vi "Modul Reset.vi"(1 "Maximale Beschleunigung":i32=500 min=0 max=2047 step=1, 2 "Mikro-Schrittweite":i32=6 min=0 max=6 step=1, 3 "maximale Positionierungsgeschwindigkeit":i32=115 min=0 max=2047 step=1, 4 "maximaler Strom [mA]":i32=700 min=0 max=1500 step=1, 5 "flow control":u16(ring) items=["None"=0, "XON/XOFF"=1, "RTS/CTS"=2, "DTR/DSR"=4], 6 "VISA resource name":refnum<visa-resource-name>="COM5", 7 "stop bits":u16(ring)=10 items=["1.0"=10, "1.5"=15, "2.0"=20], 8 "parity":u16(ring) items=["None", "Odd", "Even", "Mark", "Space"], 9 "data bits":u16=8 min=5 max=8 step=1, 10 "baud rate":u32=9600) -> (0 "Fehler":bool)   [LabVIEW 2019]
doc: "Die VI \"Modul Reset\" schickt eine Reihe von Befehlen an das Modul TMCM-110 das an eine Serielle Schnittstelle angeschlossen sein muss. Diese setzen und speichern die werte für:\n-maximale Positioniergeschwindigkeit\n-Mikro-Schrittweite\n-maximale Beschleunigung\n-maximaler Strom [mA]\nDie Werte für den Motor sind für die Verwendung mit dem Drehmagnetometer voreingestellt und müssen daher nicht notwendigerweise beschrieben werden.\nEs ist nur darauf zu achten, dass die Adresse der seriellen RS232 Schnittstelle korrekt ist."
uses:
  <vilib>/Instr/_visa.llb/VISA Configure Serial Port (Serial Instr).vi
panel:
  out "Value":string="00"
  out "Motor":string="00"
  out "Instruction":string="1E"
  out "Data to write":string="011E01000020"
  out "Type":string="01"
  # "Durch das Durchführen dieser VI wird die aktuelle Motorposition mit der Nullposition belegt.\nDes weiteren werden die Werte für die Schrittweite und die Positionierungsgeschwindigkeit\nüberschrieben und gespeichert.\nIm Frontpanel müssen nur die Werte für die Serielle Schnittstelle korrekt eingegben werden."
  # "Daten für Schnittstelle"
  # "Daten, die an den Motor geschickt werden (live)"
  # "In den Motor zu schreibende Daten"
  # "Leuchtet diese Lampe auf kann der Motor nicht ausgelesen werden!\nFolgende Ursachen sind möglich:\n-Motor hat keinen Strom\n-Motor ist nicht angeschlossen\n-RS232 Konfigurationen sind falsch"
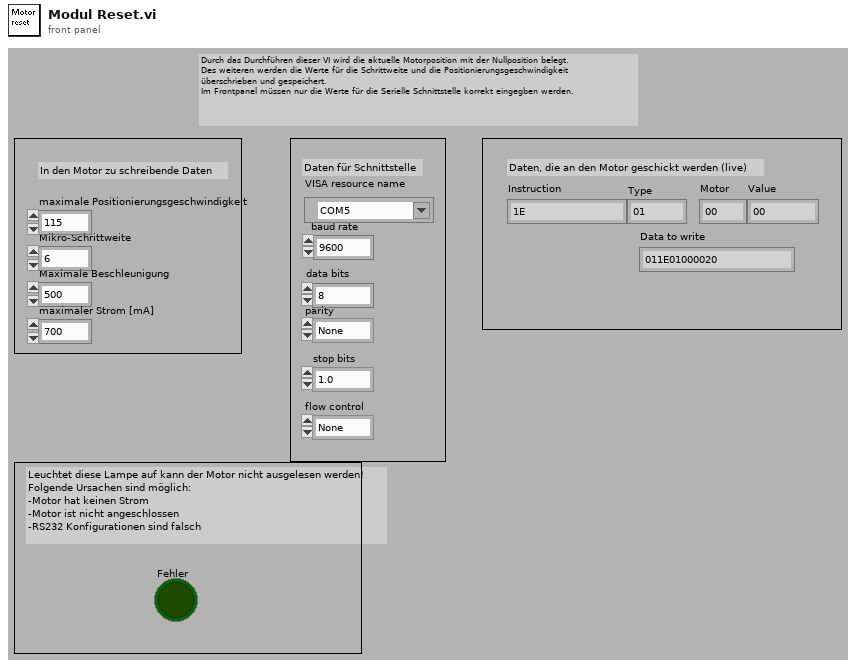
[diagram p1: front panel]
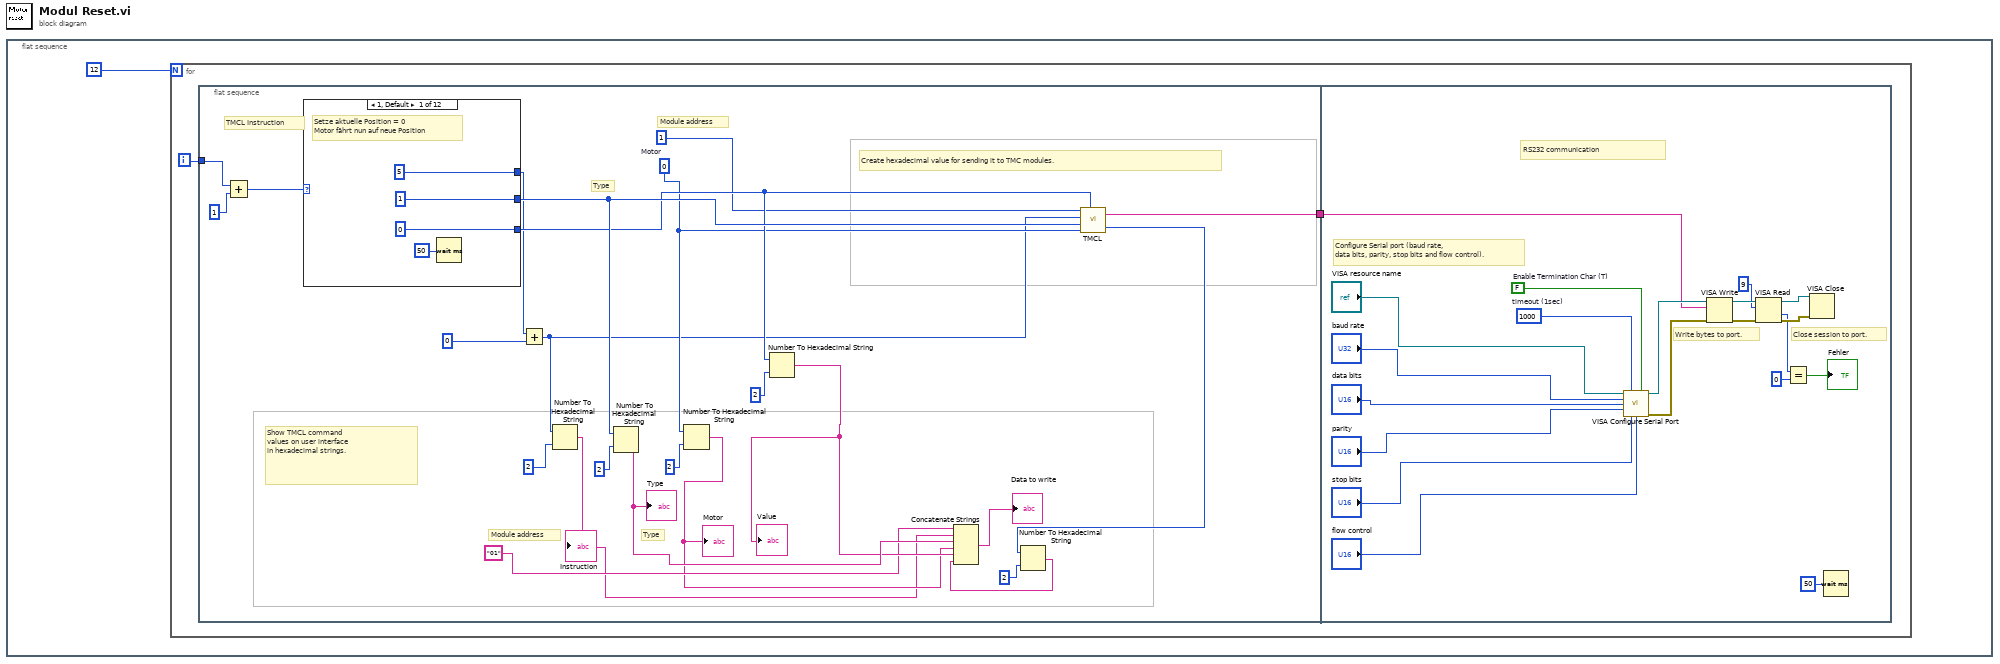
[diagram p0: block diagram]
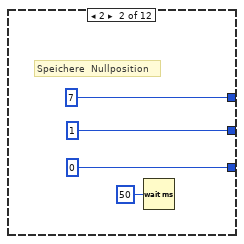
[diagram p2: hidden frame]
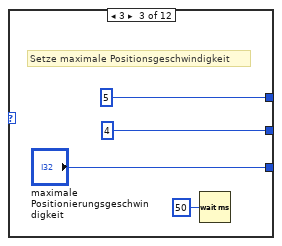
[diagram p3: hidden frame]
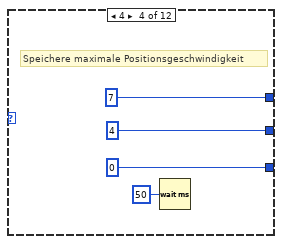
[diagram p4: hidden frame]
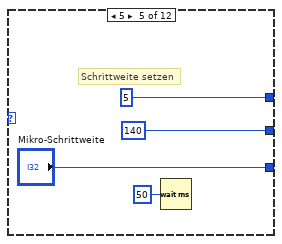
[diagram p5: hidden frame]
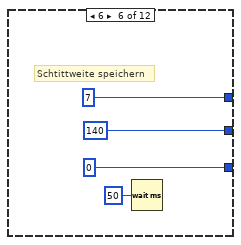
[diagram p6: hidden frame]
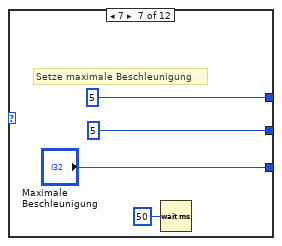
[diagram p7: hidden frame]
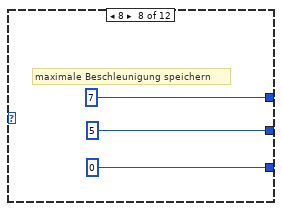
[diagram p8: hidden frame]
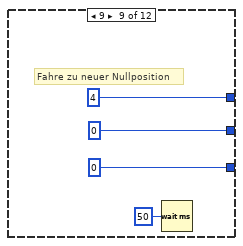
[diagram p9: hidden frame]
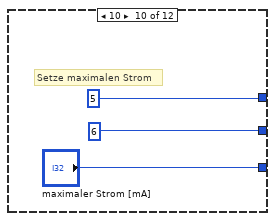
[diagram p10: hidden frame]
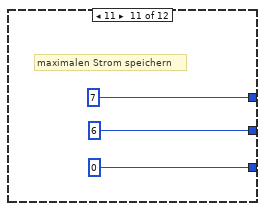
[diagram p11: hidden frame]
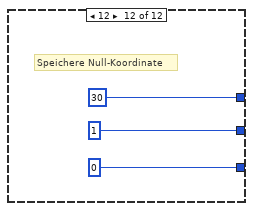
[diagram p12: hidden frame]
diagram:
  n1 = flat-sequence {
    frame #0 {
      n2 = for {
        N: 12 -> [_]
        i -> [w3]
        n3 = flat-sequence {
          tunnel: w3 -> [w5]
          tunnel: [w4] -> w2
          tunnel: w2 -> [w81]
          frame #0 {
            w21 = 0  # Motor
            # "TMCL Instruction"
            # "Type"
            # "Create hexadecimal value for sending it to TMC modules."
            # "Show TMCL command\nvalues on user interface\nin hexadecimal strings."
            # "Type"
            # "Module address"
            # "Module address"
            n4 = Add(x=w5, y=1) -> (x+y=w26:i32)
            n5 = case shown="1, Default" w26 {
              tunnel: [5 7 5 7 5 7 5 7 4 5 7 30] -> w20
              tunnel: [1 1 4 4 140 140 5 5 0 6 6 1] -> w24
              tunnel: [0 0 "maximale Positionierungsgeschwindigkeit" 0 "Mikro-Schrittweite" 0 "Maximale Beschleunigung" 0 0 "maximaler Strom [mA]" 0 0] -> w22
              frame 1, Default {
                # "Setze aktuelle Position = 0\nMotor fährt nun auf neue Position"
                n6 = Wait (ms)(milliseconds to wait=u32 50 ("Zu wartende ms")) -> ()  [unwired: 1 out]
              }
              frame 2 {
                # "Speichere  Nullposition"
                n7 = Wait (ms)(milliseconds to wait=u32 50 ("Zu wartende ms")) -> ()  [unwired: 1 out]
              }
              frame 3 {
                # "Setze maximale Positionsgeschwindigkeit"
                n8 = Wait (ms)(milliseconds to wait=u32 50 ("Zu wartende ms")) -> ()  [unwired: 1 out]
              }
              frame 4 {
                # "Speichere maximale Positionsgeschwindigkeit"
                n9 = Wait (ms)(milliseconds to wait=u32 50 ("Zu wartende ms")) -> ()  [unwired: 1 out]
              }
              frame 5 {
                # "Schrittweite setzen"
                n10 = Wait (ms)(milliseconds to wait=u32 50 ("Zu wartende ms")) -> ()  [unwired: 1 out]
              }
              frame 6 {
                # "Schtittweite speichern"
                n11 = Wait (ms)(milliseconds to wait=u32 50 ("Zu wartende ms")) -> ()  [unwired: 1 out]
              }
              frame 7 {
                # "Setze maximale Beschleunigung"
                n12 = Wait (ms)(milliseconds to wait=u32 50 ("Zu wartende ms")) -> ()  [unwired: 1 out]
              }
              frame 8 {
                # "maximale Beschleunigung speichern"
              }
              frame 9 {
                # "Fahre zu neuer Nullposition"
                n13 = Wait (ms)(milliseconds to wait=u32 50 ("Zu wartende ms")) -> ()  [unwired: 1 out]
              }
              frame 10 {
                # "Setze maximalen Strom"
              }
              frame 11 {
                # "maximalen Strom speichern"
              }
              frame 12 {
                # "Speichere Null-Koordinate"
              }
            }
            n14 = Add(x=w20, y=0) -> (x+y=w15:i32)
            n15 = Number To Hexadecimal String(1:2, 2:w15) -> (0:w8:string)
            "Instruction" <- w8
            n16 = Number To Hexadecimal String(1:2, 2:w24) -> (0:w25:string)
            "Type" <- w25
            n17 = Number To Hexadecimal String(1:2, 2:w21) -> (0:w11:string)
            "Motor" <- w11
            n18 = Number To Hexadecimal String(1:2, 2:w22) -> (0:w18:string)
            "Value" <- w18
            n19 = call "TMCL.vi"("Address"=1, "Instruction"=w15, "Type"=w24, "Motor"=w21, "Value"=w22) -> ("Hexadecimal value"=w4:string, "CRC (Optional)"=w19:i32)
            n20 = Number To Hexadecimal String(1:2, 2:w19) -> (0:w14:string)
            n21 = Concatenate Strings("01", w8, w25, w11, w18, w14) -> (→"Data to write":string)
          }
          frame #1 {
            w83 = FALSE  # Enable Termination Char (T)
            w82 = u32 1000  # timeout (1sec)
            # "RS232 communication"
            # "Write bytes to port."
            # "Configure Serial port (baud rate,\ndata bits, parity, stop bits and flow control)."
            # "Close session to port."
            n22 = call-poly "VISA Configure Serial Port"("VISA resource name"="VISA resource name", "timeout (10sec)"=w82, "Enable Termination\nChar (T)"=w83, "baud rate (9600)"="baud rate", "data bits (8)"="data bits", "parity (0:none)"="parity", "stop bits (10: 1 bit)"="stop bits", "flow control (0:none)"="flow control") -> ("VISA resource name out"=w90:refnum<visa-resource-name>, "error out"=w91:errorcluster)  [unwired: 6 in]
            n23 = VISA Write(VISA resource name=w90, write buffer=w81, error in (no error)=w91) -> (VISA resource name out=w77:refnum<visa-resource-name>, error out=w79:errorcluster)  [unwired: 1 out]
            n24 = VISA Read(VISA resource name=w77, byte count=u32 9 ("Byte-Anzahl"), error in (no error)=w79) -> (VISA resource name out=w76:refnum<visa-resource-name>, return count=w74:u32, error out=w78:errorcluster)  [unwired: 1 out]
            n25 = Equal?(x=w74, y=u32 0) -> (x = y?=→"Fehler":bool)
            n26 = VISA Close(VISA resource name=w76, error in (no error)=w78) -> ()  [unwired: 1 out]
            n27 = Wait (ms)(milliseconds to wait=u32 50 ("Zu wartende ms")) -> ()  [unwired: 1 out]
          }
        }
      }
    }
  }
